vi "Select Digitize Function.vi"(8 "error in (no error)":errorcluster, 11 "VISA resource name":refnum<visa-resource-name>) -> (0 "error out":errorcluster, 3 "VISA resource name out":refnum<visa-resource-name>)   [LabVIEW 2018, in "Keithley DMM7512.lvlib"]
doc: "This VI selects which type of digitize function is active."
uses:
  <instrlib>/Keithley DMM7512/Keithley DMM7512.lvlib
panel:
  in  "Function":u16(ring) items=["Digitize Voltage", "Digitize Current"]
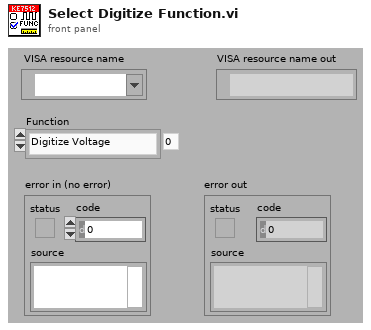
[diagram p1: front panel]
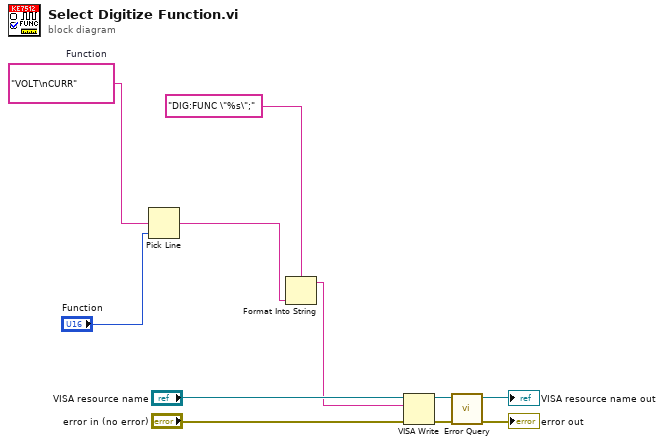
[diagram p0: block diagram]
diagram:
  w4 = "VOLT\nCURR"  # Function
  n1 = Pick Line(multi-line string=w4, line index="Function") -> (output string=w2:string)  [unwired: 1 out]
  n2 = Format Into String(format string="DIG:FUNC \"%s\";", w2) -> (resulting string=w1:string)  [unwired: 2 in, 1 out]
  n3 = VISA Write(VISA resource name="VISA resource name", write buffer=w1, error in (no error)="error in (no error)") -> (VISA resource name out=w9:refnum<visa-resource-name>, error out=w8:errorcluster)  [unwired: 1 out]
  n4 = call <instrlib>:"Error Query.vi"("error in (no error)"=w8, "VISA resource name"=w9) -> ("error out"=→"error out":errorcluster, "VISA resource name out"=→"VISA resource name out":refnum<visa-resource-name>)  [unwired: 8 out]
